vi "Post-Connect Action.vi"(8 "error in (no error)":errorcluster, 11 "Notifying Nested Endpoint in":refnum<class "Notifying Nested Endpoint.lvclass">) -> (0 "error out":errorcluster, 3 "Notifying Nested Endpoint out":refnum<class "Notifying Nested Endpoint.lvclass">)   [LabVIEW 2020, in "Notifying Nested Endpoint.lvclass"]
doc: "This override sends an Endpoint Connected message to this actor's caller.\n\nEndpoint Connected is a message of the Nested Endpoint Caller actor interface."
uses:
  Notifying Nested Endpoint.lvclass
  Nested Endpoint/Nested Endpoint/Nested Endpoint.lvclass
  Nested Endpoint Caller/Nested Endpoint Caller Messages/Endpoint Connected Msg/Endpoint Connected Msg.lvclass
  <vilib>/ActorFramework/Actor/Actor.lvclass
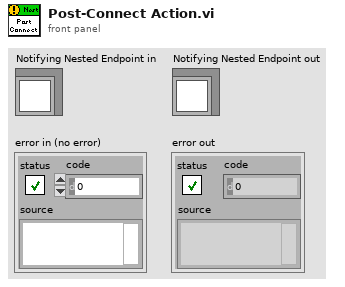
[diagram p1: front panel]
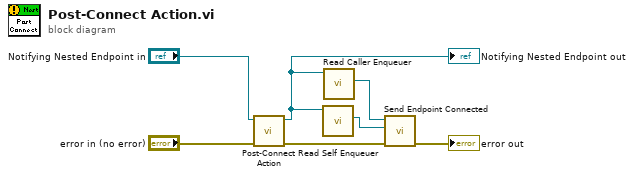
[diagram p0: block diagram]
diagram:
  n1 = call-parent "Post-Connect Action.vi"("error in (no error)"="error in (no error)", "Network Endpoint in"="Notifying Nested Endpoint in") -> ("error out"=w7:errorcluster, "Network Endpoint out"=w2:refnum<class "Notifying Nested Endpoint.lvclass">)  [unwired: 8 in]
  "Notifying Nested Endpoint out" <- w2
  n2 = call <vilib>:"Read Self Enqueuer.vi"("Actor"=w2) -> ("Self Enqueuer"=w1:refnum<class "Message Enqueuer.lvclass">)  [unwired: 10 in]
  n3 = call <vilib>:"Read Caller Enqueuer.vi"("Actor"=w2) -> ("Caller Enqueuer"=w3:refnum<class "Message Enqueuer.lvclass">)  [unwired: 10 in]
  n4 = call "Send Endpoint Connected.vi"("error in (no error)"=w7, "Endpoint"=w1, "Message Enqueuer"=w3) -> ("error out"=→"error out":errorcluster)  [unwired: 7 in, 1 out]
